vi "Super Market Billing System edit 3.123.vi"() -> ()   [LabVIEW 2021]
uses:
  <vilib>/Utility/file.llb/Write Delimited Spreadsheet (string).vi
  <vilib>/regexp/Match Regular Expression.xnode
panel:
  in  "Tab Control":enum32{"Page 1", "Page 2", "Page 3"}(tab)
  in  "adress":string
  out "Horizontal Progress Bar":u8(slide) scale=0.0..100.0
  in  "password":string
  in  "Email":string
  in  "OK Button":bool
  in  "Rise 5Kg":bool
  in  "Dal 1Kg":bool
  in  "Salt 400g":bool
  in  "Coconut Oil 1L":bool
  in  "Cilli Powder 100g":bool
  in  "Curry Powder 100g":bool
  in  "Turmeric Powder 50g":bool
  in  "Milk Powder 1kg":bool
  in  "Sugar  1kg":bool
  out "Rs.":dbl
  out "Rs.":dbl
  out "Rs.":dbl
  out "Rs.":dbl
  in  "Quantitiy":dbl min=0.0 format="%#.1f"
  out "Rs.":dbl
  in  "Quantitiy":dbl min=0.0 format="%#.1f"
  out "Rs":dbl
  in  "Quantitiy":dbl min=0.0 format="%#.1f"
  out "Rs.":dbl
  in  "Quantitiy":dbl min=0.0 format="%#.1f"
  in  "Quantitiy":dbl min=0.0 format="%#.1f"
  in  "Quantitiy":dbl min=0.0 format="%#.1f"
  in  "Quantitiy":dbl min=0.0 format="%#.1f"
  in  "Quantitiy":dbl min=0.0 format="%#.1f"
  in  "Tea 100g":bool
  in  "Quantitiy":dbl min=0.0 format="%#.1f"
  in  "Quantitiy":dbl min=0.0 format="%#.1f"
  out "Rs.":dbl
  out "Rs.":dbl
  out "Rs.":dbl
  out "Rs.":dbl
  out "Rs.":dbl
  out "Rs.":dbl
  out "Rs.":dbl
  out "Rs. 5":dbl
  out "Rs. 6":dbl
  out "Rs.":dbl
  out "Rs.":dbl
  out "Rs.":dbl
  out "Rs.":dbl
  out "Discount   Rs.":dbl format="%#.2f"
  in  "kg":dbl min=0.0 format="%#.3f"
  in  "Papaya":bool
  in  "kg":dbl min=0.0 format="%#.3f"
  in  "Graps":bool
  in  "kg":dbl min=0.0 format="%#.3f"
  in  "Orange":bool
  in  "kg":dbl min=0.0 format="%#.3f"
  in  "Apple":bool
  in  "kg":dbl min=0.0 format="%#.3f"
  in  "Banana":bool
  out "Bill   Rs.":dbl format="%#.2f"
  out "Discount percentage":string
  out "Total Bill   Rs.":dbl format="%#.2f"
  in  "kg":dbl min=0.0 format="%#.3f"
  in  "Cabege":bool
  in  "kg":dbl min=0.0 format="%#.3f"
  in  "Bringle":bool
  in  "kg":dbl min=0.0 format="%#.3f"
  in  "Beans":bool
  in  "kg":dbl min=0.0 format="%#.3f"
  in  "Leeks":bool
  in  "kg":dbl min=0.0 format="%#.3f"
  in  "Carrot":bool
  in  "stop":bool
  in  "stop 2":bool
  out "Your Bill Details":string
  in  "stop 3":bool
  # "WELCOME TO A SUPER MARCKET...."
  # "Price per 1kg (Rs.)"
  # "Quantities(kg)"
  # "Price  (Rs.)"
  # "Quantities"
  # "Vegetables"
  # "Product List"
  # "Fruits"
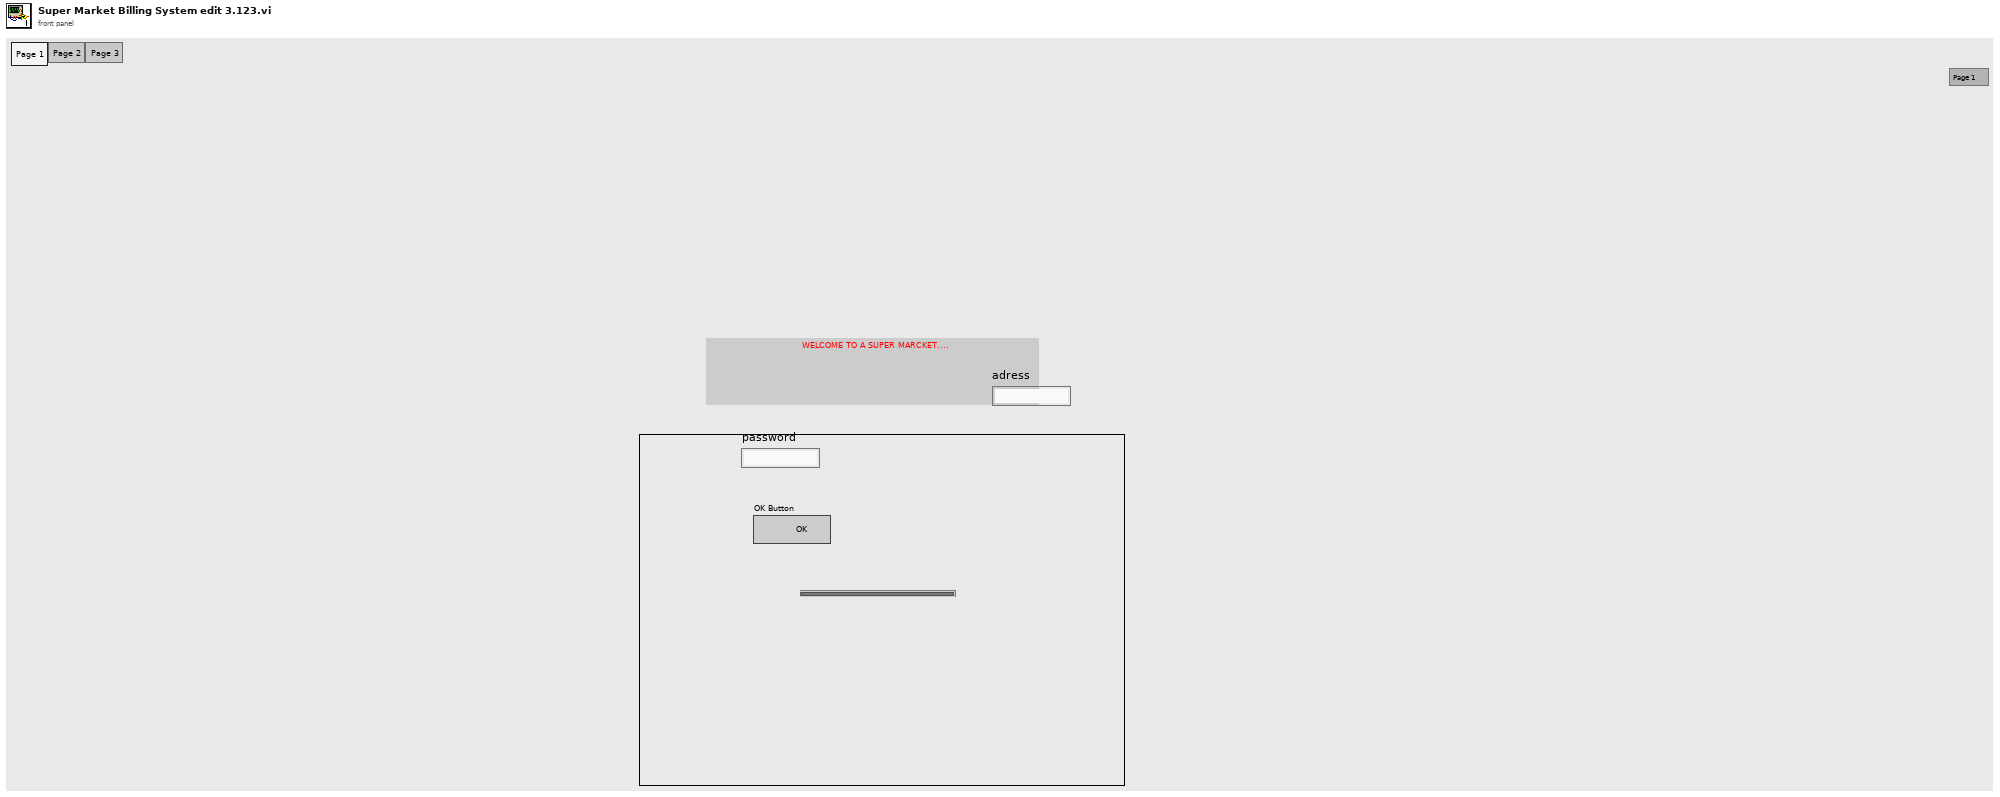
[diagram p1: front panel]
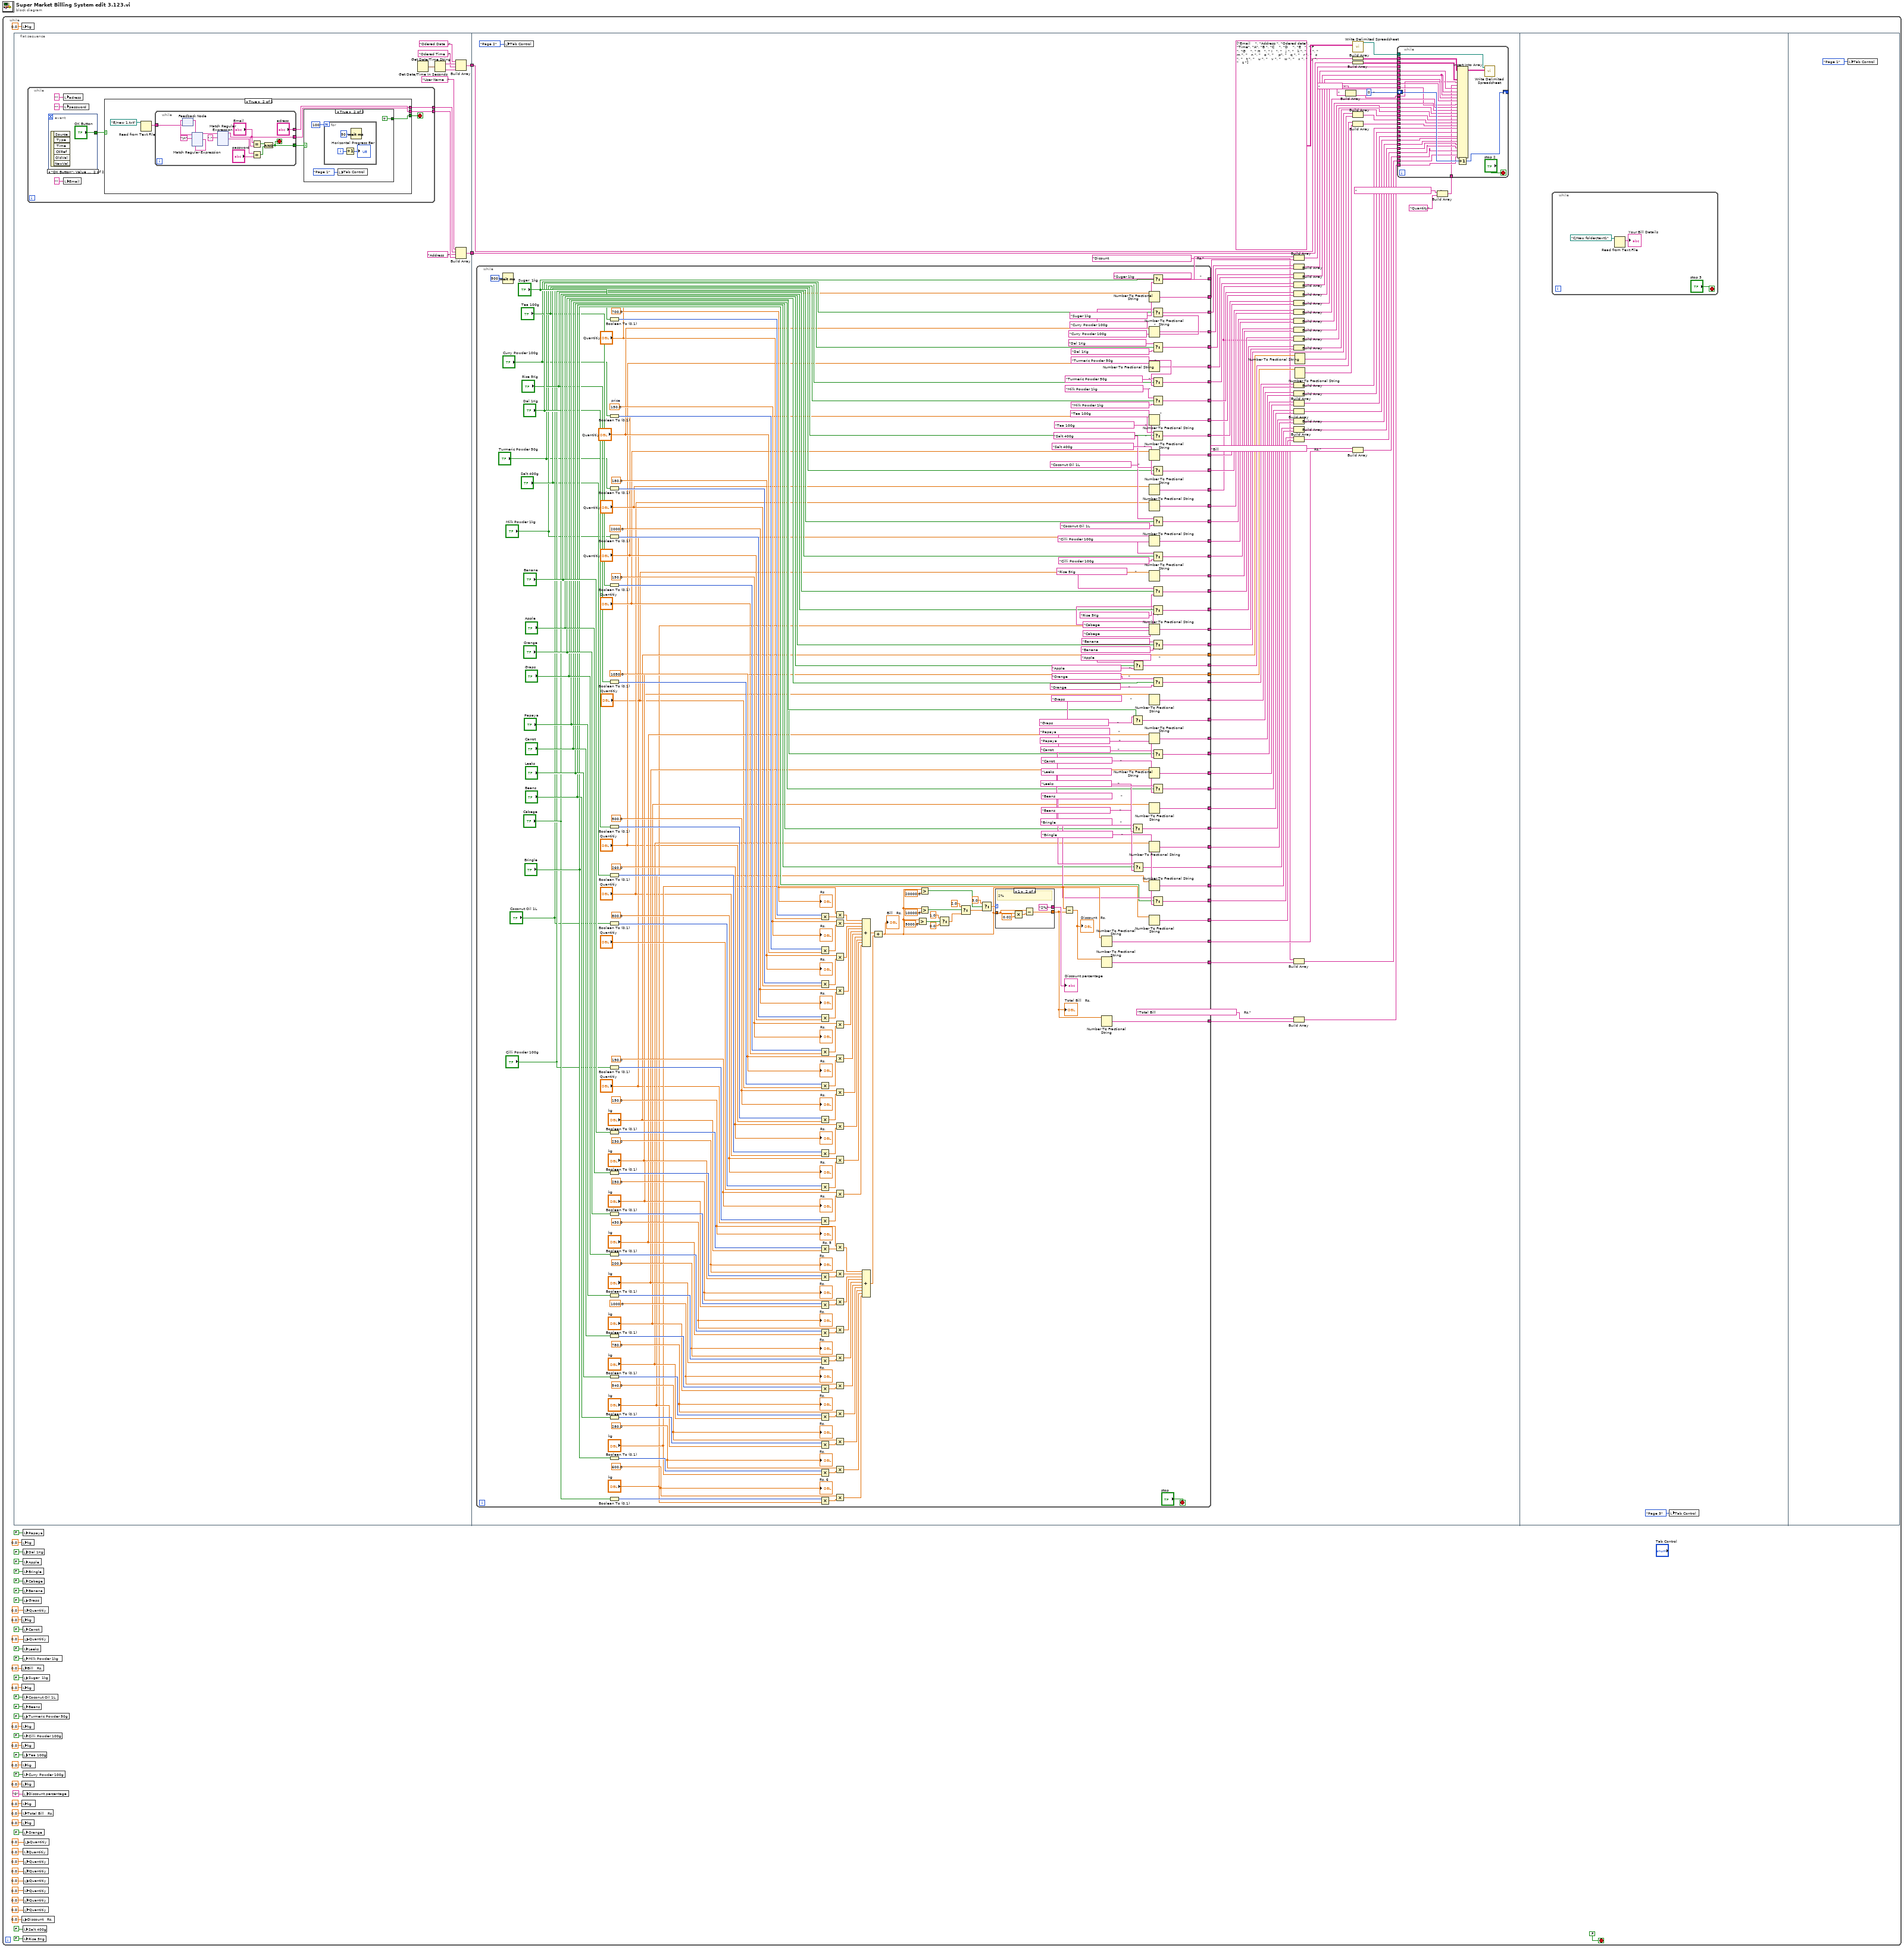
[diagram p0: block diagram]
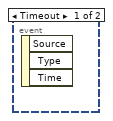
[diagram p2: hidden frame]
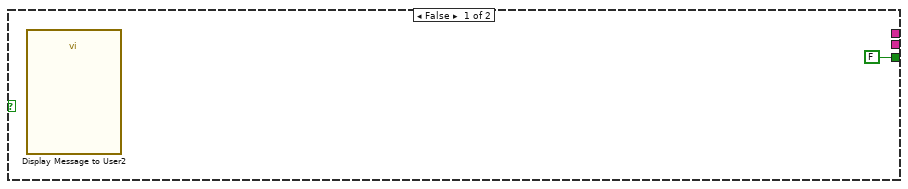
[diagram p3: hidden frame]
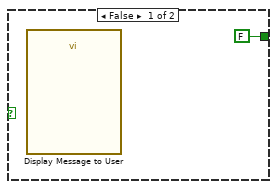
[diagram p4: hidden frame]
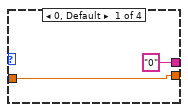
[diagram p5: hidden frame]
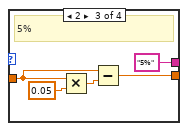
[diagram p6: hidden frame]
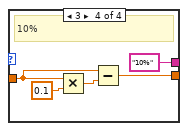
[diagram p7: hidden frame]
diagram:
  n1 = while {
    stop <- FALSE stop-if-true
    n2 = flat-sequence {
      tunnel: [w56] -> w46
      tunnel: [w48] -> w1
      tunnel: w46 -> [w412]
      tunnel: w1 -> [w338]
      frame #0 {
        n3 = while {
          tunnel: [w65] -> w52
          tunnel: [w64] -> w51
          stop <- w63 stop-if-true
          n4 = event shown="[1] \"OK Button\": Value Change" {
            selector: _ -> [_ _]
            dyn-events: _ -> [_ _]
            timeout: _ -> [_ _]
            tunnel: [_ "OK Button"] -> w59
            event Timeout {
              n5 = event-data() -> ()  [unwired: 1 in, 3 out]
            }
            event "OK Button": Value Change {
              n6 = event-data() -> ()  [unwired: 1 in, 6 out]
            }
          }
          n7 = local write "adress"("" ("adress")) -> ()
          n8 = local write "password"("" ("String 2")) -> ()
          n9 = local write "Email"("" ("String")) -> ()
          n10 = case shown="True" w59 {
            tunnel: [_ w70] -> w65
            tunnel: [_ w71] -> w64
            tunnel: [FALSE w69] -> w63
            frame False {
              n11 = call "Display Message to User2"() -> ()  [unwired: 10 in, 2 out]
            }
            frame True {
              n12 = Read from Text File(file (use dialog)=path "E:/new 1.txt") -> (text=w73:string)  [unwired: 3 in, 3 out]
              n13 = while {
                tunnel: w73 -> [w94]
                tunnel: ["adress"] -> w70
                tunnel: ["Email"] -> w71
                tunnel: [w81] -> w68
                stop <- w81 stop-if-true
                n14 = feedback #1(w94) -> (w93:string)
                n15 = xnode "Match Regular Expression"("input string"=w93, "regular expression"="\n") -> ("before match"=w90:string, "after match"=w92:string)  [unwired: 4 in, 3 out]
                n16 = feedback-in #1(w92) -> ()
                n17 = xnode "Match Regular Expression"("input string"=w90, "regular expression"=",") -> ("before match"=w87:string, "after match"=w88:string)  [unwired: 4 in, 3 out]
                n18 = Equal?(x="Email", y=w87) -> (x = y?=w85:bool)
                n19 = Equal?(x=w88, y="password") -> (x = y?=w84:bool)
                n20 = And(x=w85, y=w84) -> (x .and. y?=w81:bool)
              }
              n21 = case shown="True" w68 {
                tunnel: [FALSE TRUE] -> w69
                frame False {
                  n22 = call "Display Message to User"() -> ()  [unwired: 10 in, 2 out]
                }
                frame True {
                  n23 = for {
                    N: 100 -> [_]
                    i -> [w78]
                    n24 = Increment(x=w78) -> (x+1=→"Horizontal Progress Bar":i32)
                    n25 = Wait (ms)(milliseconds to wait=u32 50 ("millisecond timer value")) -> ()  [unwired: 1 out]
                  }
                  n26 = local write "Tab Control"(enum32{"Page 1", "Page 2"}."Page 1" ("Tab Control")) -> ()
                }
              }
            }
          }
        }
        n27 = Get Date/Time In Seconds() -> (seconds since 1Jan1904=w57:timestamp)
        n28 = Get Date/Time String(seconds (now)=w57) -> (date string=w55:string, time string=w58:string)  [unwired: 2 in]
        n29 = Build Array("Odered Date  :" ("element"), w55, "Odered Time  :" ("element"), w58) -> (w56:string[])
        n30 = Build Array("User Name  :" ("element"), w52, "Address  :" ("element"), w51) -> (w48:string[])
      }
      frame #1 {
        n31 = while {
          tunnel: [w572] -> w404
          tunnel: [w569] -> w406
          tunnel: [w568] -> w407
          tunnel: [w558] -> w370
          tunnel: [w538] -> w368
          tunnel: [w537] -> w366
          tunnel: [w528] -> w364
          tunnel: [w527] -> w362
          tunnel: [w526] -> w360
          tunnel: [w525] -> w358
          tunnel: [w524] -> w356
          tunnel: [w523] -> w354
          tunnel: [w522] -> w352
          tunnel: ["kg"] -> w411
          tunnel: ["kg"] -> w410
          tunnel: [w518] -> w365
          tunnel: [w516] -> w363
          tunnel: [w513] -> w361
          tunnel: [w512] -> w359
          tunnel: [w511] -> w357
          tunnel: [w508] -> w355
          tunnel: [w505] -> w353
          tunnel: [w504] -> w351
          tunnel: [w473] -> w403
          tunnel: [w472] -> w401
          tunnel: [w471] -> w399
          tunnel: [w470] -> w398
          tunnel: [w469] -> w396
          tunnel: [w468] -> w394
          tunnel: [w467] -> w387
          tunnel: [w466] -> w391
          tunnel: [w465] -> w389
          tunnel: [w464] -> w388
          tunnel: [w461] -> w400
          tunnel: [w460] -> w402
          tunnel: [w458] -> w385
          tunnel: [w456] -> w397
          tunnel: [w454] -> w395
          tunnel: [w449] -> w393
          tunnel: [w448] -> w392
          tunnel: [w447] -> w390
          tunnel: [w446] -> w386
          stop <- "stop" stop-if-true
          w588 = 200.0 ("price")
          w585 = 430.0 ("price")
          w582 = 250.0 ("price")
          w579 = 230.0 ("price")
          w576 = 150.0 ("price")
          w603 = 600.0 ("price")
          w600 = 280.0 ("price")
          w597 = 540.0 ("price")
          w594 = 780.0 ("price")
          w591 = 1000.0 ("price")
          w649 = 150.0 ("price")
          w646 = 700.0 ("price")
          w643 = 2000.0 ("price")
          w640 = 180.0 ("price")
          w637 = 150.0  # price
          w662 = 190.0 ("price")
          w659 = 800.0 ("price")
          w656 = 260.0 ("price")
          w654 = 500.0 ("price")
          w651 = 1050.0 ("price")
          n32 = Wait (ms)(milliseconds to wait=u32 500) -> ()  [unwired: 1 out]
          n33 = Boolean To (0,1)(Boolean="Sugar  1kg") -> (0, 1=w647:i16)
          n34 = Boolean To (0,1)(Boolean="Curry Powder 100g") -> (0, 1=w636:i16)
          n35 = Boolean To (0,1)(Boolean="Turmeric Powder 50g") -> (0, 1=w641:i16)
          n36 = Boolean To (0,1)(Boolean="Milk Powder 1kg") -> (0, 1=w642:i16)
          n37 = Boolean To (0,1)(Boolean="Tea 100g") -> (0, 1=w648:i16)
          n38 = Boolean To (0,1)(Boolean="Rise 5Kg") -> (0, 1=w567:i16)
          n39 = Boolean To (0,1)(Boolean="Dal 1Kg") -> (0, 1=w565:i16)
          n40 = Boolean To (0,1)(Boolean="Salt 400g") -> (0, 1=w655:i16)
          n41 = Boolean To (0,1)(Boolean="Coconut Oil 1L") -> (0, 1=w661:i16)
          n42 = Boolean To (0,1)(Boolean="Cilli Powder 100g") -> (0, 1=w566:i16)
          n43 = Boolean To (0,1)(Boolean="Banana") -> (0, 1=w562:i16)
          n44 = Boolean To (0,1)(Boolean="Apple") -> (0, 1=w580:i16)
          n45 = Boolean To (0,1)(Boolean="Orange") -> (0, 1=w581:i16)
          n46 = Boolean To (0,1)(Boolean="Graps") -> (0, 1=w586:i16)
          n47 = Boolean To (0,1)(Boolean="Papaya") -> (0, 1=w587:i16)
          n48 = Boolean To (0,1)(Boolean="Carrot") -> (0, 1=w590:i16)
          n49 = Boolean To (0,1)(Boolean="Leeks") -> (0, 1=w595:i16)
          n50 = Boolean To (0,1)(Boolean="Beans") -> (0, 1=w596:i16)
          n51 = Boolean To (0,1)(Boolean="Bringle") -> (0, 1=w601:i16)
          n52 = Boolean To (0,1)(Boolean="Cabege") -> (0, 1=w602:i16)
          n53 = Multiply(x=w647, y="Quantitiy") -> (x*y=w645:dbl)
          n54 = Multiply(x=w636, y="Quantitiy") -> (x*y=w638:dbl)
          n55 = Multiply(x=w641, y="Quantitiy") -> (x*y=w639:dbl)
          n56 = Multiply(x=w642, y="Quantitiy") -> (x*y=w644:dbl)
          n57 = Multiply(x=w648, y="Quantitiy") -> (x*y=w650:dbl)
          n58 = Multiply(x=w567, y="Quantitiy") -> (x*y=w652:dbl)
          n59 = Multiply(x=w565, y="Quantitiy") -> (x*y=w653:dbl)
          n60 = Multiply(x=w655, y="Quantitiy") -> (x*y=w657:dbl)
          n61 = Multiply(x=w661, y="Quantitiy") -> (x*y=w658:dbl)
          n62 = Multiply(x=w566, y="Quantitiy") -> (x*y=w663:dbl)
          n63 = Multiply(x=w562, y="kg") -> (x*y=w577:dbl)
          n64 = Multiply(x=w580, y="kg") -> (x*y=w578:dbl)
          n65 = Multiply(x=w581, y="kg") -> (x*y=w583:dbl)
          n66 = Multiply(x=w586, y="kg") -> (x*y=w584:dbl)
          n67 = Multiply(x=w587, y="kg") -> (x*y=w589:dbl)
          n68 = Multiply(x=w590, y="kg") -> (x*y=w592:dbl)
          n69 = Multiply(x=w595, y="kg") -> (x*y=w593:dbl)
          n70 = Multiply(x=w596, y="kg") -> (x*y=w598:dbl)
          n71 = Multiply(x=w601, y="kg") -> (x*y=w599:dbl)
          n72 = Multiply(x=w602, y="kg") -> (x*y=w604:dbl)
          n73 = Multiply(x=w646, y=w645) -> (x*y=w445:dbl)
          n74 = Multiply(x=w637, y=w638) -> (x*y=w564:dbl)
          n75 = Multiply(x=w640, y=w639) -> (x*y=w635:dbl)
          n76 = Multiply(x=w643, y=w644) -> (x*y=w634:dbl)
          n77 = Multiply(x=w649, y=w650) -> (x*y=w633:dbl)
          n78 = Multiply(x=w651, y=w652) -> (x*y=w632:dbl)
          n79 = Multiply(x=w654, y=w653) -> (x*y=w631:dbl)
          n80 = Multiply(x=w656, y=w657) -> (x*y=w630:dbl)
          n81 = Multiply(x=w659, y=w658) -> (x*y=w629:dbl)
          n82 = Multiply(x=w662, y=w663) -> (x*y=w628:dbl)
          n83 = Multiply(x=w576, y=w577) -> (x*y=w563:dbl)
          n84 = Multiply(x=w579, y=w578) -> (x*y=w619:dbl)
          n85 = Multiply(x=w582, y=w583) -> (x*y=w620:dbl)
          n86 = Multiply(x=w585, y=w584) -> (x*y=w621:dbl)
          n87 = Multiply(x=w588, y=w589) -> (x*y=w622:dbl)
          n88 = Multiply(x=w591, y=w592) -> (x*y=w623:dbl)
          n89 = Multiply(x=w594, y=w593) -> (x*y=w624:dbl)
          n90 = Multiply(x=w597, y=w598) -> (x*y=w625:dbl)
          n91 = Multiply(x=w600, y=w599) -> (x*y=w626:dbl)
          n92 = Multiply(x=w603, y=w604) -> (x*y=w627:dbl)
          n93 = Compound Arithmetic op=ADD(w445, w564, w635, w634, w633, w632, w631, w630, w629, w628) -> (w575:dbl)
          n94 = Compound Arithmetic op=ADD(w563, w619, w620, w621, w622, w623, w624, w625, w626, w627) -> (w574:dbl)
          n95 = Compound Arithmetic op=ADD(w575, w574) -> (w573:dbl)
          "Bill   Rs." <- w573
          n96 = Greater?(x=w573, y=5000.0) -> (0:w616:bool)
          n97 = Greater?(x=w573, y=20000.0) -> (0:w618:bool)
          n98 = Greater?(x=w573, y=10000.0) -> (0:w617:bool)
          n99 = Select(t=1.0, s=w616, f=0.0) -> (s? t:f=w612:dbl)
          n100 = Select(t=2.0, s=w617, f=w612) -> (s? t:f=w613:dbl)
          n101 = Select(t=3.0, s=w618, f=w613) -> (s? t:f=w614:dbl)
          n102 = case shown="1" w614 {
            tunnel: [w666 w670 w673 w678] -> w571
            tunnel: w573 -> [w666 w669 w674 w679]
            tunnel: ["0" ("discount") "2%" ("discount") "5%" ("discount") "10%" ("discount")] -> w615
            frame 0, Default {
            }
            frame 1 {
              # "2%"
              n103 = Multiply(x=w669, y=0.02) -> (x*y=w667:dbl)
              n104 = Subtract(x=w669, y=w667) -> (x-y=w670:dbl)
            }
            frame 2 {
              # "5%"
              n105 = Multiply(x=w674, y=0.05) -> (x*y=w675:dbl)
              n106 = Subtract(x=w674, y=w675) -> (x-y=w673:dbl)
            }
            frame 3 {
              # "10%"
              n107 = Multiply(x=w679, y=0.1) -> (x*y=w680:dbl)
              n108 = Subtract(x=w679, y=w680) -> (x-y=w678:dbl)
            }
          }
          "Total Bill   Rs." <- w571
          "Discount percentage" <- w615
          n109 = Subtract(x=w573, y=w571) -> (x-y=w570:dbl)
          "Discount   Rs." <- w570
          n110 = Number To Fractional String(number=w573) -> (F-format string=w572:string)  [unwired: 3 in]
          n111 = Number To Fractional String(number=w570) -> (F-format string=w568:string)  [unwired: 3 in]
          n112 = Number To Fractional String(number=w571) -> (F-format string=w569:string)  [unwired: 3 in]
          n113 = Select(t="Leeks                                                       ", s="Leeks", f="Leeks                                                      ") -> (s? t:f=w525:string)
          n114 = Select(t="Graps                                                      " ("f"), s="Graps", f="Graps                                                       ") -> (s? t:f=w528:string)
          n115 = Select(t="Apple                                                      ", s="Apple", f="Apple                                                      ") -> (s? t:f=w538:string)
          n116 = Select(t="Beans                                                       ", s="Beans", f="Beans                                                      ") -> (s? t:f=w524:string)
          n117 = Number To Fractional String(number="Quantitiy") -> (F-format string=w460:string)  [unwired: 3 in]
          n118 = Number To Fractional String(number="Quantitiy") -> (F-format string=w461:string)  [unwired: 3 in]
          n119 = Number To Fractional String(number="Quantitiy") -> (F-format string=w446:string)  [unwired: 3 in]
          n120 = Number To Fractional String(number="Quantitiy") -> (F-format string=w456:string)  [unwired: 3 in]
          n121 = Number To Fractional String(number="Quantitiy") -> (F-format string=w454:string)  [unwired: 3 in]
          n122 = Number To Fractional String(number="Quantitiy") -> (F-format string=w458:string)  [unwired: 3 in]
          n123 = Number To Fractional String(number="Quantitiy") -> (F-format string=w449:string)  [unwired: 3 in]
          n124 = Number To Fractional String(number="Quantitiy") -> (F-format string=w448:string)  [unwired: 3 in]
          n125 = Number To Fractional String(number="Quantitiy") -> (F-format string=w447:string)  [unwired: 3 in]
          n126 = Number To Fractional String(number="kg") -> (F-format string=w504:string)  [unwired: 3 in]
          n127 = Number To Fractional String(number="kg") -> (F-format string=w518:string)  [unwired: 3 in]
          n128 = Number To Fractional String(number="kg") -> (F-format string=w516:string)  [unwired: 3 in]
          n129 = Number To Fractional String(number="kg") -> (F-format string=w513:string)  [unwired: 3 in]
          n130 = Number To Fractional String(number="kg") -> (F-format string=w512:string)  [unwired: 3 in]
          n131 = Number To Fractional String(number="kg") -> (F-format string=w511:string)  [unwired: 3 in]
          n132 = Number To Fractional String(number="kg") -> (F-format string=w508:string)  [unwired: 3 in]
          n133 = Number To Fractional String(number="kg") -> (F-format string=w505:string)  [unwired: 3 in]
          n134 = Select(t="Suger 1kg                                                       ", s="Sugar  1kg", f="Suger 1kg                                                       ") -> (s? t:f=w473:string)
          n135 = Select(t="Curry Powder 100g                                       ", s="Curry Powder 100g", f="Curry Powder 100g                                       ") -> (s? t:f=w472:string)
          n136 = Select(t="Dal 1Kg                                                           ", s="Dal 1Kg", f="Dal 1Kg                                                           ") -> (s? t:f=w464:string)
          n137 = Select(t="Turmeric Powder 50g                                   ", s="Turmeric Powder 50g", f="Turmeric Powder 50g                                   ") -> (s? t:f=w471:string)
          n138 = Select(t="Milk Powder 1kg                                           ", s="Milk Powder 1kg", f="Milk Powder 1kg                                           ") -> (s? t:f=w470:string)
          n139 = Select(t="Tea 100g                                                          ", s="Tea 100g", f="Tea 100g                                                           ") -> (s? t:f=w469:string)
          n140 = Select(t="Salt 400g                                                            ", s="Salt 400g", f="Salt 400g                                                            ") -> (s? t:f=w468:string)
          n141 = Select(t="Coconut Oil 1L                                                 ", s="Coconut Oil 1L", f="Coconut Oil 1L                                                      ") -> (s? t:f=w467:string)
          n142 = Select(t="Cilli Powder 100g                                                       ", s="Cilli Powder 100g", f="Cilli Powder 100g                                                      ") -> (s? t:f=w466:string)
          n143 = Select(t="Rise 5Kg                                                  ", s="Rise 5Kg", f="Rise 5Kg                                                 ") -> (s? t:f=w465:string)
          n144 = Select(t="Cabege                                                ", s="Cabege", f="Cabege                                                 ") -> (s? t:f=w522:string)
          n145 = Select(t="Banana                                                  ", s="Banana", f="Banana                                                   ") -> (s? t:f=w558:string)
          n146 = Select(t="Orange                                                   ", s="Orange", f="Orange                                                    ") -> (s? t:f=w537:string)
          n147 = Select(t="Papaya                                                    ", s="Papaya", f="Papaya                                                    ") -> (s? t:f=w527:string)
          n148 = Select(t="Carrot                                                      ", s="Carrot", f="Carrot                                                       ") -> (s? t:f=w526:string)
          n149 = Select(t="Bringle                                                      ", s="Bringle", f="Bringle                                                      ") -> (s? t:f=w523:string)
          "Rs." <- w651
          "Rs." <- w654
          "Rs." <- w656
          "Rs." <- w659
          "Rs." <- w662
          "Rs." <- w637
          "Rs." <- w640
          "Rs." <- w643
          "Rs" <- w646
          "Rs." <- w649
          "Rs." <- w591
          "Rs." <- w594
          "Rs." <- w597
          "Rs." <- w600
          "Rs. 6" <- w603
          "Rs. 5" <- w576
          "Rs." <- w579
          "Rs." <- w582
          "Rs." <- w585
          "Rs." <- w588
        }
        n150 = local write "Tab Control"(enum32{"Page 1", "Page 2"}."Page 2" ("Tab Control")) -> ()
        n151 = Build Array(w403, w402) -> (w380:string[])
        n152 = Build Array(w401, w400) -> (w379:string[])
        n153 = Build Array(w388, w386) -> (w371:string[])
        n154 = Build Array(w399, w385) -> (w378:string[])
        n155 = Build Array(w398, w397) -> (w377:string[])
        n156 = Build Array(w396, w395) -> (w376:string[])
        n157 = Build Array(w394, w393) -> (w375:string[])
        n158 = Build Array(w387, w392) -> (w374:string[])
        n159 = Build Array(w391, w390) -> (w373:string[])
        n160 = Build Array(w389, w385) -> (w372:string[])
        n161 = Build Array(w352, w351) -> (w341:string[])
        n162 = Build Array(w366, w365) -> (w348:string[])
        n163 = Build Array(w364, w363) -> (w347:string[])
        n164 = Build Array(w362, w361) -> (w346:string[])
        n165 = Build Array(w360, w359) -> (w345:string[])
        n166 = Build Array(w358, w357) -> (w344:string[])
        n167 = Build Array(w356, w355) -> (w343:string[])
        n168 = Build Array(w354, w353) -> (w342:string[])
        n169 = Build Array("Dicount                                                                          Rs." ("element"), w407) -> (w382:string[])
        n170 = Build Array("Total Bill                                                                          Rs." ("element"), w406) -> (w381:string[])
        n171 = Number To Fractional String(number=w411) -> (F-format string=w369:string)  [unwired: 3 in]
        n172 = Number To Fractional String(number=w410) -> (F-format string=w367:string)  [unwired: 3 in]
        n173 = Build Array("                            ", "                    " ("element")) -> (w333:string[])
        n174 = call-poly <vilib>:"Write Delimited Spreadsheet.vi"("2D data"=string[][] [["Email    "], ["Address "], ["Odered date"], ["Time"], ["A"], ["B "], ["C    "], ["D    "], ["E   "], [" F   "], ["G    "], [" H   "], [" I   "], ["   j "], ["   k "], ["   l "], ["   m "], ["   n "], ["   o "], ["    p"], ["   q "], ["   r "], ["   s "], ["   t "], ["   u "], ["   v "], ["   w "], ["   x "], ["   y "], ["   z "]] ("delimiter (\\t)")) -> ("new file path (Not A Path if cancelled)"=w408:path)  [unwired: 13 in, 1 out]
        n175 = Build Array(w412) -> (w384:string[][])
        n176 = Build Array(w338) -> (w337:string[][])
        n177 = Build Array(w370, w369) -> (w350:string[])
        n178 = Build Array(w368, w367) -> (w349:string[])
        n179 = Build Array("Bill                                                                                Rs." ("element"), w404) -> (w383:string[])
        n180 = Build Array("                                                                      " ("element"), "Quantity" ("element")) -> (w330:string[])
        n181 = while {
          tunnel: w408 -> [w443]
          shift-right: [w440] -> _
          shift-left: 0 -> [w441]
          tunnel: w384 -> [w439]
          tunnel: w383 -> [w434]
          tunnel: w382 -> [w435]
          tunnel: w381 -> [w436]
          tunnel: w380 -> [_]
          tunnel: w379 -> [w415]
          tunnel: w378 -> [w417]
          tunnel: w377 -> [w418]
          tunnel: w376 -> [w419]
          tunnel: w375 -> [w420]
          tunnel: w374 -> [w421]
          tunnel: w373 -> [w422]
          tunnel: w372 -> [w423]
          tunnel: w371 -> [w416]
          tunnel: w350 -> [w425]
          tunnel: w349 -> [w426]
          tunnel: w348 -> [w427]
          tunnel: w347 -> [w428]
          tunnel: w346 -> [w429]
          tunnel: w345 -> [w430]
          tunnel: w344 -> [w431]
          tunnel: w343 -> [w432]
          tunnel: w342 -> [w433]
          tunnel: w341 -> [w424]
          tunnel: w337 -> [w437]
          tunnel: w333 -> [w414]
          tunnel: w330 -> [w413]
          stop <- "stop 2" stop-if-true
          n182 = Increment(x=w441) -> (x+1=w440:i32)
          n183 = Insert Into Array "Insert Into Array"(array=w439, new element #1=w437, new element #2=w414, new element #3=w413, new element #4=w415, new element #5=w416, new element #6=w416, new element #7=w417, new element #8=w418, new element #9=w419, new element #10=w420, new element #11=w421, new element #12=w422, new element #13=w423, new element #14=w424, new element #15=w425, new element #16=w426, new element #17=w427, new element #18=w428, new element #19=w429, new element #20=w430, new element #21=w431, new element #22=w432, new element #23=w433, new element #24=w434, new element #25=w435, new element #26=w436) -> (w438:string[][])  [unwired: 2 in]
          n184 = call-poly <vilib>:"Write Delimited Spreadsheet.vi"("file path (dialog if empty)"=w443, "2D data"=w438) -> ()  [unwired: 12 in, 2 out]
        }
      }
      frame #2 {
        n185 = while {
          stop <- "stop 3" stop-if-true
          n186 = Read from Text File(file (use dialog)=path "C:/New folder/text1") -> (text=→"Your Bill Details":string)  [unwired: 3 in, 3 out]
        }
        n187 = local write "Tab Control"(enum32{"Page 1", "Page 2", "Page 3"}."Page 3" ("Tab Control")) -> ()
      }
      frame #3 {
        n188 = local write "Tab Control"(enum32{"Page 1", "Page 2"}."Page 1" ("Tab Control")) -> ()
      }
    }
    n189 = local write "kg"(0.0 ("kg")) -> ()
    n190 = local write "kg"(0.0 ("kg")) -> ()
    n191 = local write "kg"(0.0 ("kg")) -> ()
    n192 = local write "Bill   Rs."(0.0 ("Bill   Rs.")) -> ()
    n193 = local write "kg"(0.0 ("kg")) -> ()
    n194 = local write "kg"(0.0 ("kg")) -> ()
    n195 = local write "kg"(0.0 ("kg")) -> ()
    n196 = local write "kg"(0.0 ("kg")) -> ()
    n197 = local write "kg"(0.0 ("kg")) -> ()
    n198 = local write "kg"(0.0 ("kg")) -> ()
    n199 = local write "Total Bill   Rs."(0.0 ("Total Bill   Rs.")) -> ()
    n200 = local write "kg"(0.0 ("kg")) -> ()
    n201 = local write "Discount   Rs."(0.0 ("Discount   Rs.")) -> ()
    n202 = local write "Papaya"(FALSE ("Papaya")) -> ()
    n203 = local write "Dal 1Kg"(FALSE ("Dal 1Kg")) -> ()
    n204 = local write "Apple"(FALSE ("Apple")) -> ()
    n205 = local write "Bringle"(FALSE ("Bringle")) -> ()
    n206 = local write "Cabege"(FALSE ("Cabege")) -> ()
    n207 = local write "Banana"(FALSE ("Banana")) -> ()
    n208 = local write "Graps"(FALSE ("Graps")) -> ()
    n209 = local write "Carrot"(FALSE ("Carrot")) -> ()
    n210 = local write "Leeks"(FALSE ("Leeks")) -> ()
    n211 = local write "Milk Powder 1kg"(FALSE ("Milk Powder 1kg")) -> ()
    n212 = local write "Sugar  1kg"(FALSE ("Sugar  1kg")) -> ()
    n213 = local write "Coconut Oil 1L"(FALSE ("Coconut Oil 1L")) -> ()
    n214 = local write "Beans"(FALSE ("Beans")) -> ()
    n215 = local write "Turmeric Powder 50g"(FALSE ("Turmeric Powder 50g")) -> ()
    n216 = local write "Cilli Powder 100g"(FALSE ("Cilli Powder 100g")) -> ()
    n217 = local write "Tea 100g"(FALSE ("Tea 100g")) -> ()
    n218 = local write "Curry Powder 100g"(FALSE ("Curry Powder 100g")) -> ()
    n219 = local write "Orange"(FALSE ("Orange")) -> ()
    n220 = local write "Salt 400g"(FALSE ("Salt 400g")) -> ()
    n221 = local write "Rise 5Kg"(FALSE ("Rise 5Kg")) -> ()
    n222 = local write "Discount percentage"("0" ("Discount percentage")) -> ()
    n223 = local write "Quantitiy"(0.0 ("Quantities")) -> ()
    n224 = local write "Quantitiy"(0.0 ("quantity 16")) -> ()
    n225 = local write "Quantitiy"(0.0 ("quantity 11")) -> ()
    n226 = local write "Quantitiy"(0.0 ("quantity 12")) -> ()
    n227 = local write "Quantitiy"(0.0 ("quantity 14")) -> ()
    n228 = local write "Quantitiy"(0.0 ("quantity 17")) -> ()
    n229 = local write "Quantitiy"(0.0 ("quantity 10")) -> ()
    n230 = local write "Quantitiy"(0.0 ("quantity 13")) -> ()
    n231 = local write "Quantitiy"(0.0 ("quantity 15")) -> ()
    n232 = local write "Quantitiy"(0.0 ("Quantities 4")) -> ()
  }
